vi "DESTROY USER EVENTS.vi"(8 "error in (no error)":errorcluster, 11 "GRAFICAR_SEÑAL_ACTUALIZABLE in":refnum<class "GRAFICAR_SEÑAL_ACTUALIZABLE.lvclass">) -> (0 "error out":errorcluster)   [LabVIEW 2019, in "GRAFICAR_SEÑAL_ACTUALIZABLE.lvlib" / "GRAFICAR_SEÑAL_ACTUALIZABLE.lvclass"]
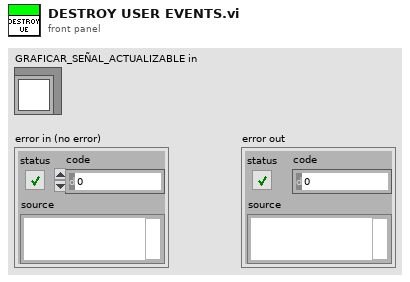
[diagram p1: front panel]
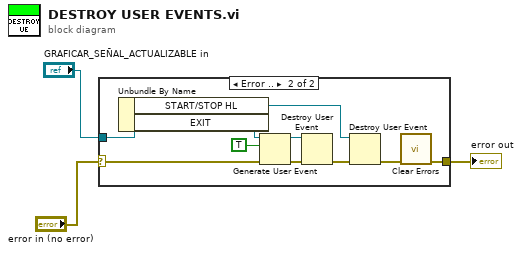
[diagram p0: block diagram]
diagram:
  n1 = case shown="Error .." "error in (no error)" {
    selector: "error in (no error)" -> [w4 w8]
    tunnel: "GRAFICAR_SEÑAL_ACTUALIZABLE in" -> [_ w14]
    tunnel: [w4 w5] -> w3
    frame No Error {
    }
    frame Error {
      n2 = Unbundle By Name(w14) -> ("START/STOP HL"=w10:refnum<user-event>, "EXIT"=w13:refnum<user-event>)
      n3 = Generate User Event(user event=w13, event data cluster=TRUE ("event data"), error in=w8) -> (user event out=w11:refnum<user-event>, error out=w12:errorcluster)  [unwired: 1 in]
      n4 = Destroy User Event(user event=w11, error in=w12) -> (error out=w9:errorcluster)
      n5 = Destroy User Event(user event=w10, error in=w9) -> (error out=w6:errorcluster)
      n6 = call <vilib>:"Clear Errors.vi"("error in (no error)"=w6) -> ("error out"=w5:errorcluster)  [unwired: 5 in, 1 out]
    }
  }
  "error out" <- w3
